vi "set or get window states.vi"(7 "old panels":T1, 8 "error in":errorcluster, 9 "set?":bool, 10 "refs":T3, 11 "Panels":T1) -> (0 "error out":errorcluster, 2 "states":T2(array[ring]), 3 "Panels out":T1)   [LabVIEW 2010]
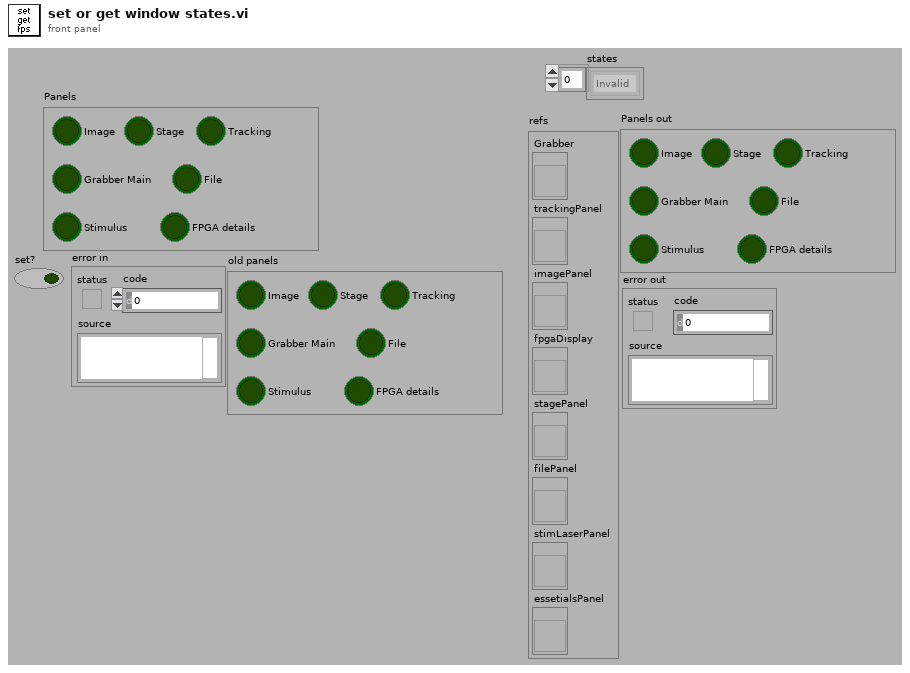
[diagram p1: front panel]
types:
  T1 = cluster{"Grabber Main":bool, "Tracking":bool, "Image":bool, "FPGA details":bool, "Stage":bool, "File":bool, "Stimulus":bool}
  T2 = enum32{"Invalid", "Standard", "Closed", "Hidden", "Minimized", "Maximized"}[]
  T3 = cluster{"Grabber":refnum<vi>, "trackingPanel":refnum<vi>, "imagePanel":refnum<vi>, "fpgaDisplay":refnum<vi>, "stagePanel":refnum<vi>, "filePanel":refnum<vi>, "stimLaserPanel":refnum<vi>, "essetialsPanel":refnum<vi>}
  T4 = enum32{"Invalid", "Standard", "Closed", "Hidden", "Minimized", "Maximized"}
  T5 = cluster{"[0]":bool, "[1]":bool, "[2]":bool, "[3]":bool, "[4]":bool, "[5]":bool, "[6]":bool}
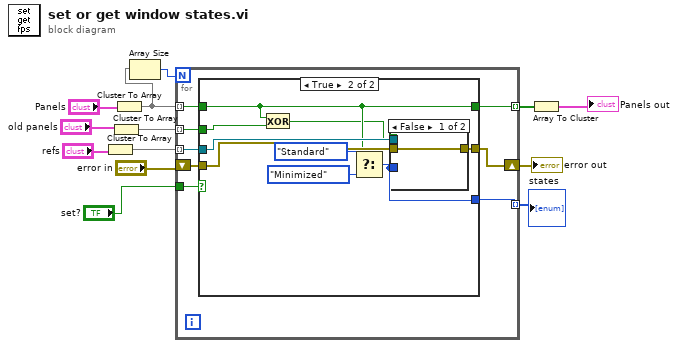
[diagram p0: block diagram]
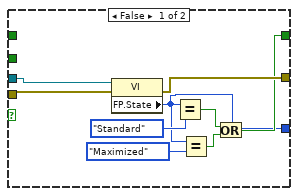
[diagram p2: hidden frame]
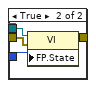
[diagram p3: hidden frame]
diagram:
  n1 = Cluster To Array(cluster="refs") -> (array=w11:refnum<vi>[])
  n2 = Cluster To Array(cluster="old panels") -> (array=w1:bool[])
  n3 = Cluster To Array(cluster="Panels") -> (array=w10:bool[])
  n4 = Array Size(array=w10) -> (size(s)=w9:i32)
  n5 = for {
    N: w9 -> [_]
    tunnel: w10 -> [w19] mode=indexing
    tunnel: w11 -> [w20] mode=indexing
    tunnel: "set?" -> [w21]
    shift-right: [w18] -> w4
    shift-left: "error in" -> [w17]
    tunnel: [w16] -> w7 mode=indexing
    tunnel: [w15] -> w3 mode=indexing
    tunnel: w1 -> [w14] mode=indexing
    n6 = case shown="True" w21 {
      tunnel: w20 -> [w30 w34]
      tunnel: w19 -> [_ w32]
      tunnel: [w29 w37] -> w18
      tunnel: w17 -> [w28 w36]
      tunnel: [w23 w32] -> w16
      tunnel: [w22 w35] -> w15
      tunnel: w14 -> [_ w33]
      frame False {
        n7 = property class="VI"(reference=w30, error in=w28) -> (error out=w29:errorcluster, "FP.State"=w22:T4)  [unwired: 1 out]
        n8 = Equal?(x=w22, y=T4."Standard") -> (x = y?=w24:bool)
        n9 = Equal?(x=w22, y=T4."Maximized") -> (x = y?=w25:bool)
        n10 = Or(x=w24, y=w25) -> (x .or. y?=w23:bool)
      }
      frame True {
        n11 = Exclusive Or(1:w33, 2:w32) -> (0:w31:bool)
        n12 = Select(t=T4."Standard" ("Front Panel Window:State"), s=w32, f=T4."Minimized" ("Front Panel Window:State")) -> (s? t:f=w35:T4)
        n13 = case shown="False" w31 {
          tunnel: [w40 w44] -> w37
          tunnel: w36 -> [w40 w43]
          tunnel: w35 -> [_ w42]
          tunnel: w34 -> [_ w41]
          frame False {
          }
          frame True {
            n14 = property class="VI"(reference=w41, error in=w43, "FP.State"=w42) -> (error out=w44:errorcluster)  [unwired: 1 out]
          }
        }
      }
    }
  }
  "error out" <- w4
  "states" <- w3
  n15 = Array To Cluster(array=w7) -> (cluster=→"Panels out":T5)
